vi "SetFootnoteReference.vi"(8 "error in (no error)":errorcluster, 10 "LvMarkdown.lvlib:FootnoteReference.lvclass":refnum<class "FootnoteReference.lvclass">, 11 "Footnote in":refnum<class "Footnote.lvclass">) -> (0 "error out":errorcluster, 3 "Footnote out":refnum<class "Footnote.lvclass">)   [LabVIEW 2021, in "LvMarkdown.lvlib" / "Footnote.lvclass"]
uses:
  Footnote.lvclass
  Footnote.lvclass/Footnote.ctl
  FootnoteReference/FootnoteReference.lvclass
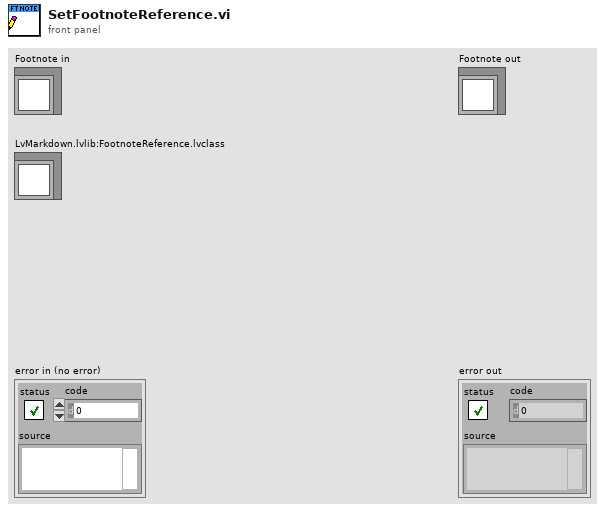
[diagram p1: front panel]
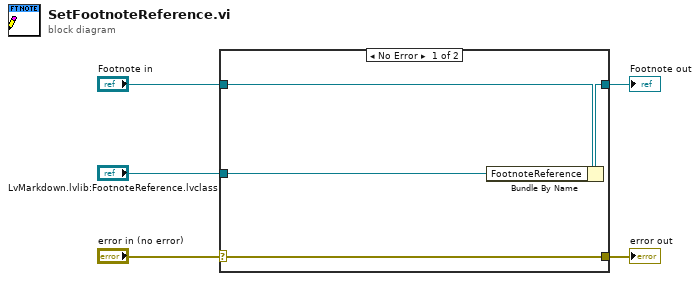
[diagram p0: block diagram]
diagram:
  n1 = case shown="No Error" "error in (no error)" {
    selector: "error in (no error)" -> [w9 w10]
    tunnel: [w9 w10] -> w4
    tunnel: [w7 w11] -> w2
    tunnel: "Footnote in" -> [w8 w11]
    tunnel: "LvMarkdown.lvlib:FootnoteReference.lvclass" -> [w6 _]
    frame No Error {
      n2 = Bundle By Name(cluster=w8, "FootnoteReference"=w6) -> (w7:refnum<class "Footnote.lvclass">)
    }
    frame Error {
    }
  }
  "error out" <- w4
  "Footnote out" <- w2
